vi "Generate Data Frame Vectors.vi"(0 "RFFE RegRead Command in":refnum<class "RFFE RegRead Command.lvclass">, 11 "error in (no error)":errorcluster) -> (4 "RFFE RegRead Command out":refnum<class "RFFE RegRead Command.lvclass">, 6 "Data Frame Vectors":string[](array[string]), 15 "error out":errorcluster)   [LabVIEW 2018, in "MIPI RFFE API.lvlib" / "RFFE RegRead Command.lvclass"]
uses:
  RFFE RegRead Command.lvclass
  MIPI RFFE API.lvlib
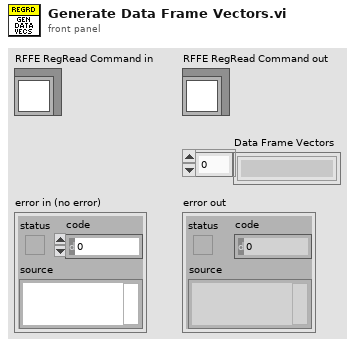
[diagram p1: front panel]
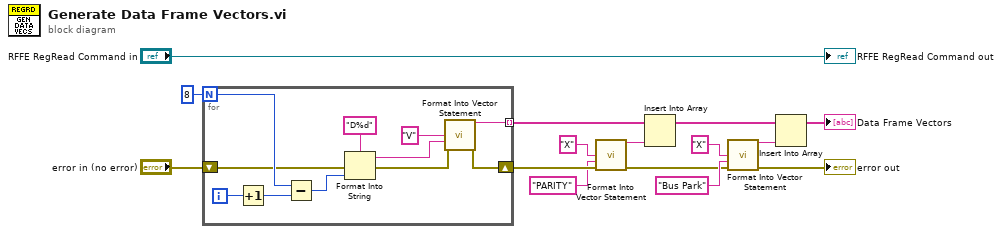
[diagram p0: block diagram]
diagram:
  n1 = for {
    N: 8 -> [w23]
    shift-right: [w26] -> w12
    shift-left: "error in (no error)" -> [w20]
    tunnel: [w24] -> w11 mode=indexing
    i -> [w22]
    n2 = Increment(x=w22) -> (x+1=w21:i32)
    n3 = Subtract(x=w23, y=w21) -> (x-y=w18:i32)
    n4 = Format Into String(format string="D%d", error in=w20, w18) -> (resulting string=w17:string, error out=w19:errorcluster)  [unwired: 1 in]
    n5 = call "Format Into Vector Statement.vi"("DATA (0)"="V", "Comment"=w17, "error in (no error)"=w19) -> ("Vector Statement"=w24:string, "error out"=w26:errorcluster)  [unwired: 11 in]
  }
  n6 = call "Format Into Vector Statement.vi"("DATA (0)"="X", "Comment"="PARITY", "error in (no error)"=w12) -> ("Vector Statement"=w10:string, "error out"=w5:errorcluster)  [unwired: 11 in]
  n7 = Insert Into Array(array=w11, new element=w10) -> (w3:string[])  [unwired: 1 in]
  n8 = call "Format Into Vector Statement.vi"("DATA (0)"="X", "Comment"="Bus Park", "error in (no error)"=w5) -> ("Vector Statement"=w4:string, "error out"=→"error out":errorcluster)  [unwired: 11 in]
  n9 = Insert Into Array(array=w3, new element=w4) -> (→"Data Frame Vectors":string[])  [unwired: 1 in]
  "RFFE RegRead Command out" <- "RFFE RegRead Command in"
